vi "Config.vi"(8 "error in (no error)":errorcluster, 10 "Setting":variant, 11 "Chroma190020 HiPOT in":refnum<class "Chroma190020 HiPOT.lvclass">) -> (0 "error out":errorcluster, 3 "Chroma190020 HiPOT out":refnum<class "Chroma190020 HiPOT.lvclass">)   [LabVIEW 2019, in "Concrete.lvlib" / "Chroma190020 HiPOT.lvclass"]
uses:
  Chroma190020 HiPOT.lvclass
  Chroma190020 HiPOT.lvclass/Chroma190020 HiPOT.ctl
panel:
  in  "Real Setting":T1={"dc voltage"=100, "high limit"=4e-07, "test time(s)"=3.0, "Channel"=""} {"high limit" format="%#_10f"}
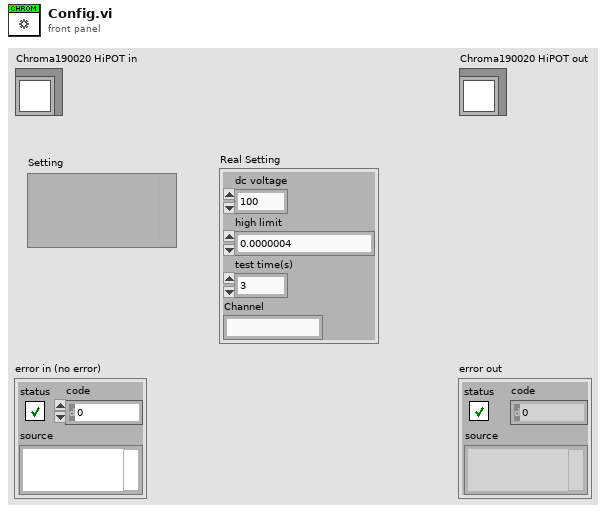
[diagram p1: front panel]
types:
  T1 = cluster{"dc voltage":i32, "high limit":dbl, "test time(s)":dbl, "Channel":string}
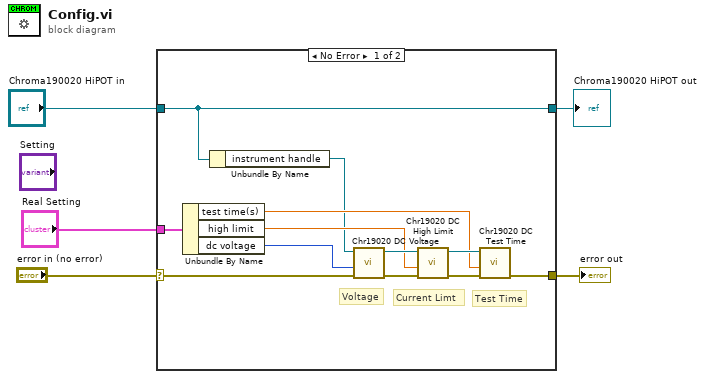
[diagram p0: block diagram]
diagram:
  n1 = case shown="No Error" "error in (no error)" {
    selector: "error in (no error)" -> [w12 w19]
    tunnel: [w11 w19] -> w4
    tunnel: [w6 w18] -> w2
    tunnel: "Chroma190020 HiPOT in" -> [w6 w18]
    tunnel: "Real Setting" -> [w17 _]
    frame No Error {
      # "Current Limt"
      # "Test Time"
      # "Voltage"
      n2 = Unbundle By Name(w17) -> ("test time(s)"=w8:dbl, "high limit"=w9:dbl, "dc voltage"=w10:i32)
      n3 = Unbundle By Name(w6) -> ("instrument handle"=w7:refnum<k15>)
      n4 = call <instrlib>:"Chr19020 DC Voltage.vi"("error in (no error)"=w12, "dc voltage"=w10, "instrument handle"=w7) -> ("error out"=w15:errorcluster, "instrument handle out"=w16:refnum<k15>)  [unwired: 7 in]
      n5 = call <instrlib>:"Chr19020 DC High Limit.vi"("error in (no error)"=w15, "high limit"=w9, "instrument handle"=w16) -> ("error out"=w13:errorcluster, "instrument handle out"=w14:refnum<k15>)  [unwired: 7 in]
      n6 = call <instrlib>:"Chr19020 DC Test Time.vi"("error in (no error)"=w13, "test time"=w8, "instrument handle"=w14) -> ("error out"=w11:errorcluster)  [unwired: 7 in, 1 out]
    }
    frame Error {
    }
  }
  "error out" <- w4
  "Chroma190020 HiPOT out" <- w2
